vi "Acquisition Message Loop.vi"(8 "error in (no error)":errorcluster, 9 "queue out":refnum<queue>, 10 "Data Notifier":refnum<notifier>, 11 "Message Queues":T1) -> (0 "error out":errorcluster)   [LabVIEW 2018, in "Acquisition.lvlib"]
doc: "Message loop for handling messages pertaining to the acquisition of data from the hardware."
uses:
  Acquisition.lvlib
  support/Message Queue/Message Queue.lvlib
  Acquisition State.ctl
  support/Message Queue/Enqueue Message (Single).vi
  <vilib>/ErrorRing/Error Ring.xnode
  GlobalVariable/GlobalPowerByTime.vi
  GlobalVariable/Globalt0.vi
  GlobalVariable/GlobalLongueurOnde.vi
  GlobalVariable/GlobalDisconnected.vi
  GlobalVariable/GlobalPosXbyTime.vi
  GlobalVariable/GlobalPosYbyTime.vi
  GlobalVariable/GlobalProfileByTime.vi
  GlobalVariable/GlobalTimeStep.vi
  GlobalVariable/GlobalFirstRep.vi
  GlobalVariable/GlobalTensionByTime.vi
  GlobalVariable/GlobalTemperatureByTime.vi
  <vilib>/Utility/error.llb/Error Cluster From Error Code.vi
  support/Message Queue/Message Cluster.ctl
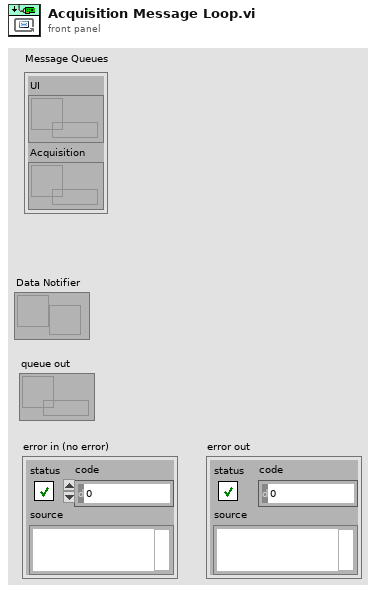
[diagram p1: front panel]
types:
  T1 = cluster{"UI":refnum<queue>, "Acquisition":refnum<queue>}
  T2 = typedef "Acquisition.lvlib/Acquisition State.ctl" = enum16{"Idle", "Acquiring"}
  T3 = enum16{"open", "replace", "create", "open or create", "replace or create", "replace or create with confirmation"}
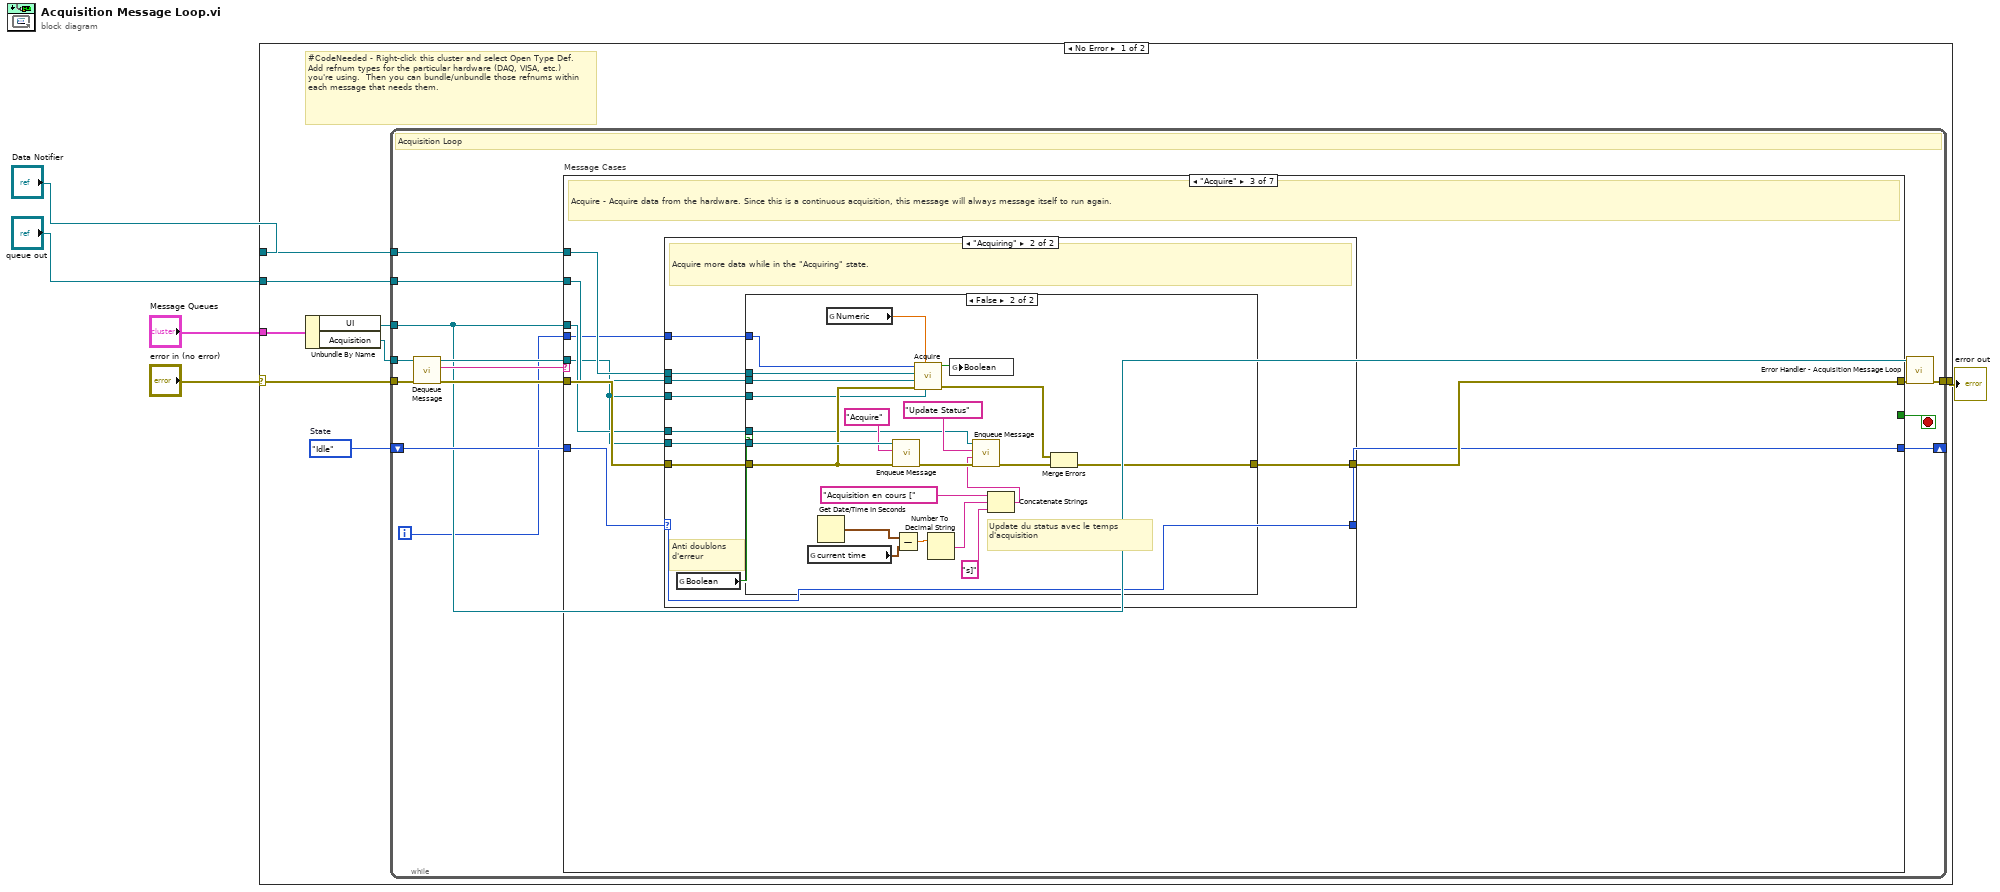
[diagram p0: block diagram]
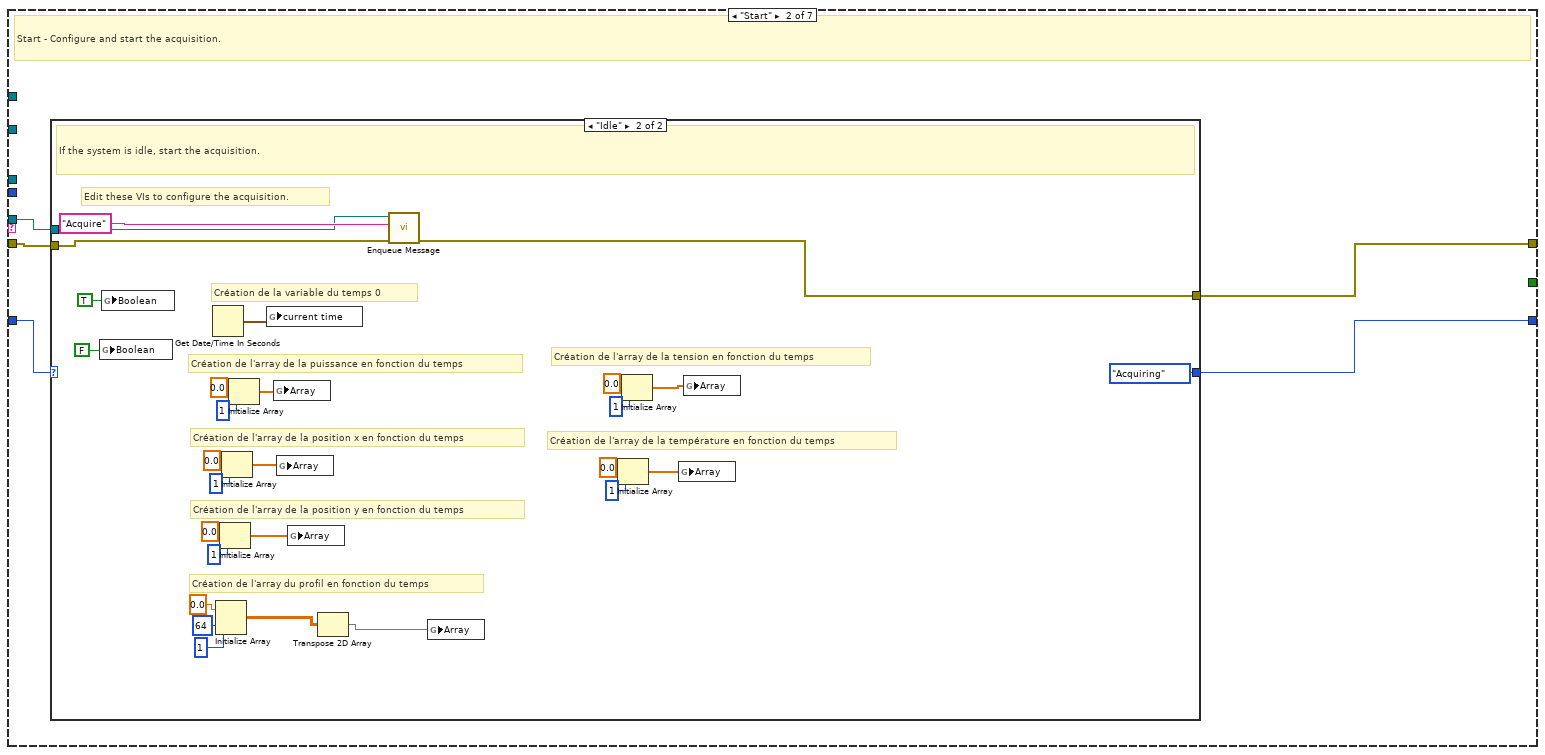
[diagram p3: hidden frame]
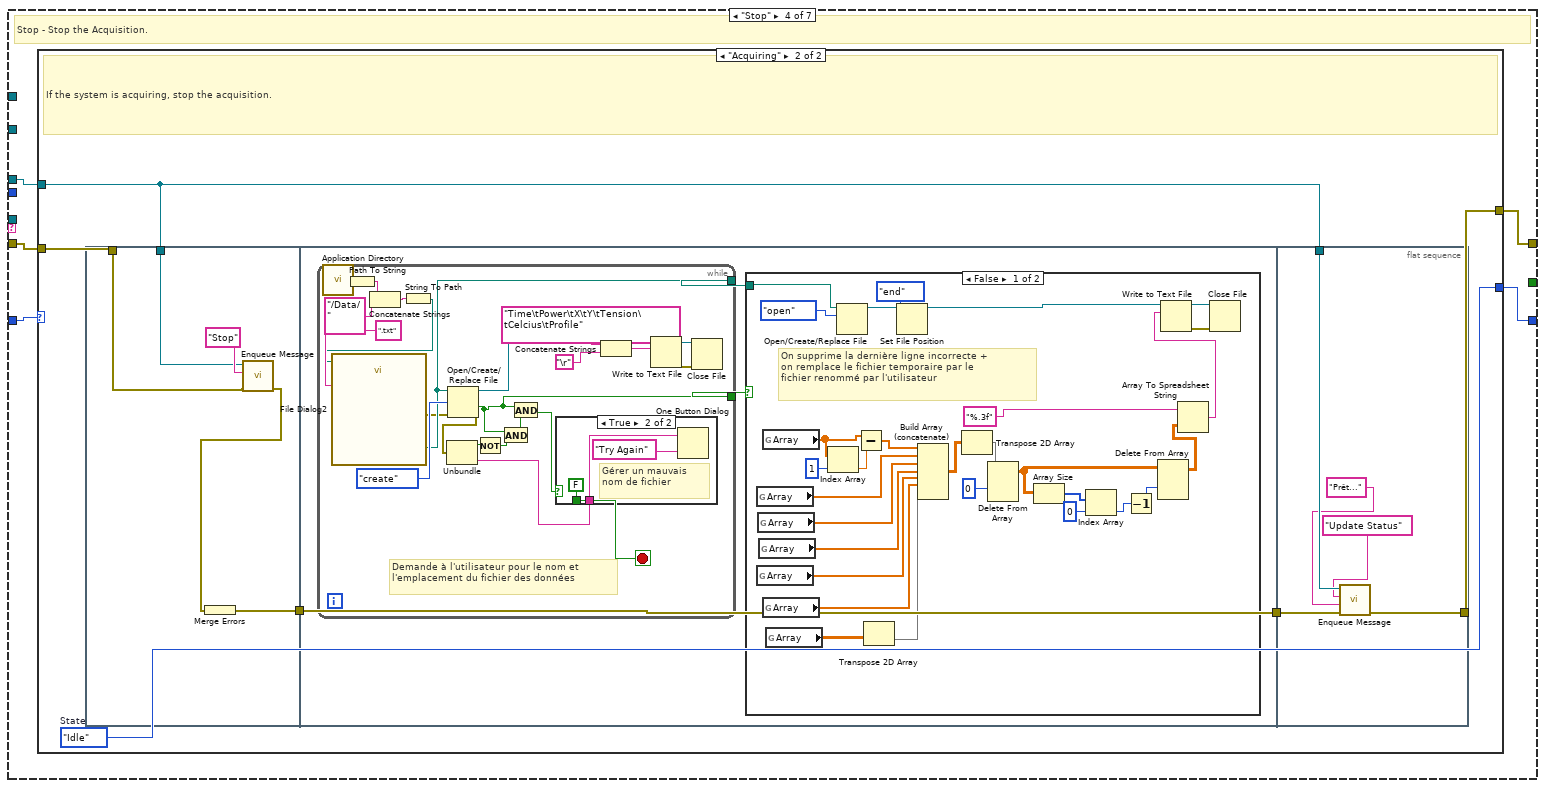
[diagram p7: hidden frame]
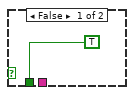
[diagram p10: hidden frame]
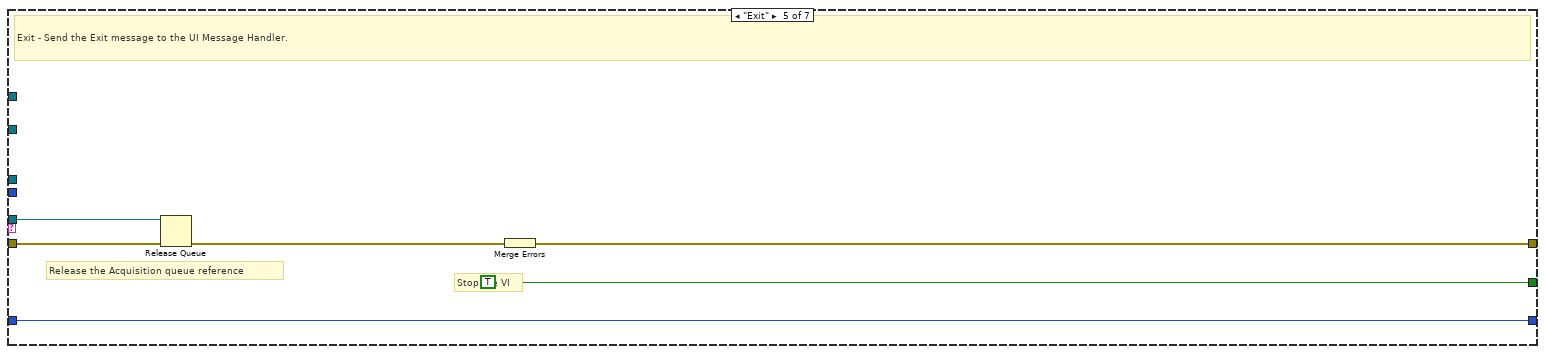
[diagram p11: hidden frame]
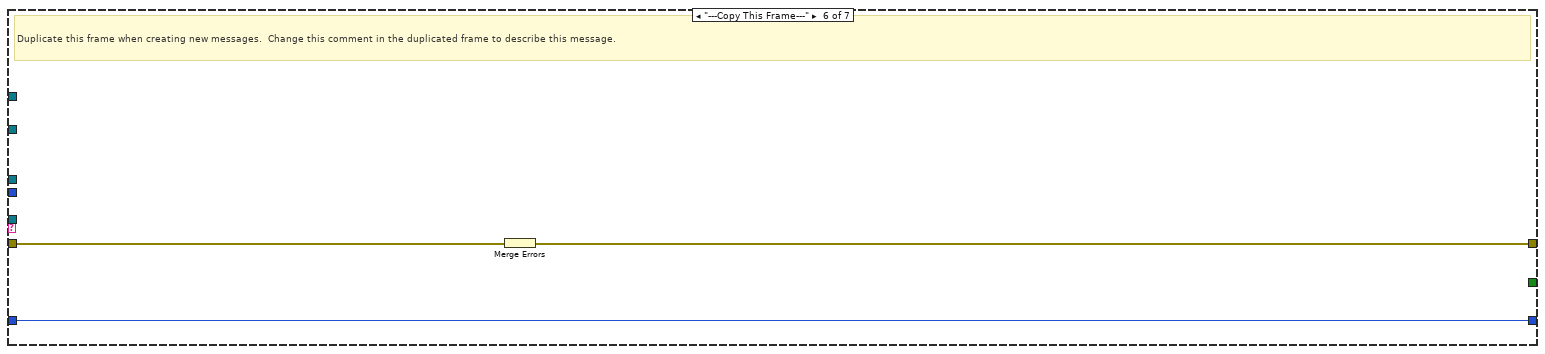
[diagram p12: hidden frame]
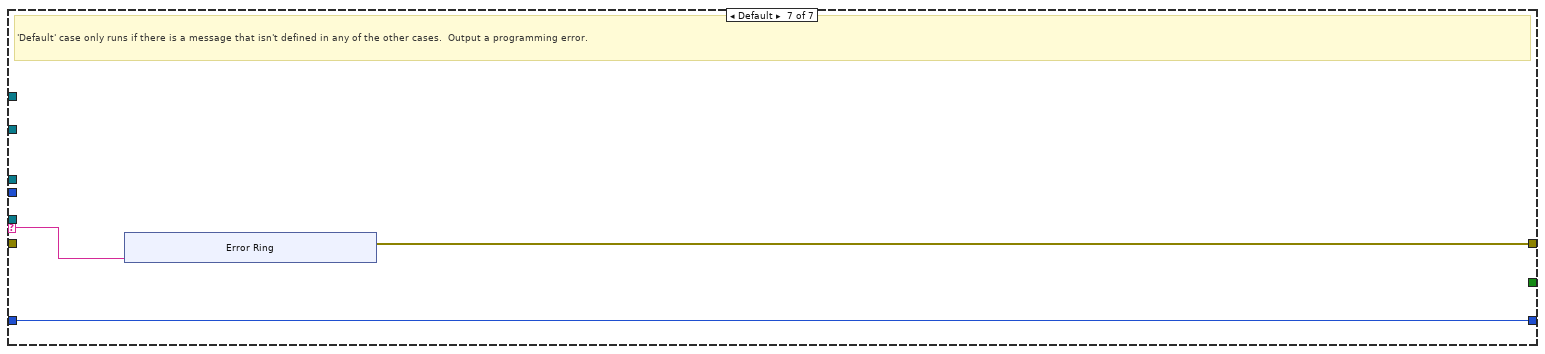
[diagram p13: hidden frame]
diagram:
  n1 = case shown="No Error" "error in (no error)" {
    selector: "error in (no error)" -> [w10 w210]
    tunnel: "Message Queues" -> [w13 _]
    tunnel: [w11 w210] -> w4
    tunnel: "Data Notifier" -> [w8 _]
    tunnel: "queue out" -> [w7 _]
    frame No Error {
      w6 = Acquisition_State."Idle"  # State
      # "#CodeNeeded - Right-click this cluster and select Open Type Def.  Add refnum types for the particular hardware (DAQ, VISA, etc.) you're using.  Then you can bundle/unbundle those refnums within each message that needs them."
      n2 = Unbundle By Name(w13) -> ("UI"=w9:refnum<queue>, "Acquisition"=w12:refnum<queue>)
      n3 = while {
        tunnel: w12 -> [w15]
        tunnel: w9 -> [w16]
        tunnel: w8 -> [w23]
        tunnel: w7 -> [w22]
        shift-right: [w20] -> _
        shift-left: w6 -> [w21]
        tunnel: w10 -> [w26]
        tunnel: [w19] -> w11
        i -> [w14]
        stop <- w27 stop-if-true
        # "Acquisition Loop"
        n4 = call "Dequeue Message.vi"("error in (no error)"=w26, "Message Queue"=w15) -> ("error out"=w25:errorcluster, "Message"=w24:string, "dup Message Queue"=w17:refnum<queue>)  [unwired: 6 in, 1 out]
        n5 = case "Message Cases" shown="\"Acquire\"" w24 {
          selector: w24 -> [_ _ _ _ _ _ w200]
          tunnel: w17 -> [_ w32 w66 _ w192 _ _]
          tunnel: w25 -> [w29 w33 w72 w112 w194 w199 _]
          tunnel: [w29 w34 w73 w110 w195 w198 w201] -> w18
          tunnel: [_ _ _ _ TRUE _ _] -> w27
          tunnel: w16 -> [_ _ w67 w111 _ _ _]
          tunnel: w23 -> [_ _ w71 _ _ _ _]
          tunnel: w22 -> [_ _ w70 _ _ _ _]
          tunnel: w21 -> [w28 w30 w68 w113 w191 w197 w202]
          tunnel: [w28 w31 w69 w109 w191 w197 w202] -> w20
          tunnel: w14 -> [_ _ w65 _ _ _ _]
          frame "Initialize" {
            # "Initialize  - Initialize is currently a no-op.  The hardware initialization takes place in the 'Start' message."
          }
          frame "Start" {
            # "Start - Configure and start the acquisition."
            n6 = case shown="\"Idle\"" w30 {
              selector: w30 -> [w35 _]
              tunnel: [w36 w60] -> w34
              tunnel: w33 -> [w36 w64]
              tunnel: w32 -> [_ w61]
              tunnel: [w35 Acquisition_State."Acquiring" ("Acquisition State")] -> w31
              frame "Acquiring" {
                # "The system is already acquiring. Ignore the \"Start\" message."
              }
              frame "Idle" {
                # "Création de l'array de la température en fonction du temps"
                # "Création de l'array de la tension en fonction du temps"
                # "Création de la variable du temps 0"
                # "Création de l'array du profil en fonction du temps"
                # "Création de l'array de la position y en fonction du temps"
                # "Création de l'array de la position x en fonction du temps"
                # "Création de l'array de la puissance en fonction du temps"
                # "Edit these VIs to configure the acquisition."
                # "If the system is idle, start the acquisition."
                n7 = global write "GlobalDisconnected.vi" "Boolean"(FALSE) -> ()
                n8 = global write "GlobalFirstRep.vi" "Boolean"(TRUE ("Boolean")) -> ()
                n9 = Get Date/Time In Seconds() -> (seconds since 1Jan1904=w43:timestamp)
                n10 = Initialize Array(0.0, 64 ("dimension size"), 1 ("dimension size")) -> (w56:dbl[][])
                n11 = Initialize Array(0.0, 1) -> (w57:dbl[])
                n12 = Initialize Array(0.0, 1) -> (w58:dbl[])
                n13 = Initialize Array(0.0, 1) -> (w59:dbl[])
                n14 = global write "Globalt0.vi" "current time"(w43) -> ()
                n15 = global write "GlobalPowerByTime.vi" "Array"(w59) -> ()
                n16 = global write "GlobalPosXbyTime.vi" "Array"(w58) -> ()
                n17 = global write "GlobalPosYbyTime.vi" "Array"(w57) -> ()
                n18 = Transpose 2D Array(2D array=w56) -> (transposed array=w55:dbl[][])
                n19 = call-poly "Enqueue Message.vi"("error in (no error)"=w64, "Message"="Acquire", "Message Queue"=w61) -> ("error out"=w60:errorcluster)  [unwired: 7 in, 1 out]
                n20 = global write "GlobalProfileByTime.vi" "Array"(w55) -> ()
                n21 = Initialize Array(0.0, 1) -> (w37:dbl[])
                n22 = Initialize Array(0.0, 1) -> (w38:dbl[])
                n23 = global write "GlobalTemperatureByTime.vi" "Array"(w37) -> ()
                n24 = global write "GlobalTensionByTime.vi" "Array"(w38) -> ()
              }
            }
          }
          frame "Acquire" {
            # "Acquire - Acquire data from the hardware. Since this is a continuous acquisition, this message will always message itself to run again."
            n25 = case shown="\"Acquiring\"" w68 {
              selector: w68 -> [w74 w81]
              tunnel: [w75 w85] -> w73
              tunnel: w66 -> [_ w84]
              tunnel: w72 -> [w75 w80]
              tunnel: w71 -> [_ w83]
              tunnel: w70 -> [_ w82]
              tunnel: [w74 w81] -> w69
              tunnel: w67 -> [_ w79]
              tunnel: w66 -> [_ w78]
              tunnel: w65 -> [_ w76]
              frame "Idle" {
                # "Ignore \"Acquire\" messages when the acquisition is idle."
              }
              frame "Acquiring" {
                # "Anti doublons\nd'erreur"
                # "Acquire more data while in the \"Acquiring\" state."
                n26 = global read "GlobalDisconnected.vi" "Boolean"() -> (w77:bool)
                n27 = case shown="False" w77 {
                  tunnel: [w86 w108] -> w85
                  tunnel: w84 -> [_ w107]
                  tunnel: w83 -> [_ w104]
                  tunnel: w82 -> [_ w103]
                  tunnel: w80 -> [w86 w102]
                  tunnel: w79 -> [_ w91]
                  tunnel: w78 -> [_ w90]
                  tunnel: w76 -> [_ w87]
                  frame True {
                  }
                  frame False {
                    # "Update du status avec le temps\nd'acquisition"
                    n28 = global read "Globalt0.vi" "current time"() -> (w97:timestamp)
                    n29 = Get Date/Time In Seconds() -> (seconds since 1Jan1904=w96:timestamp)
                    n30 = global read "GlobalLongueurOnde.vi" "Numeric"() -> (w89:dbl)
                    n31 = call-poly "Enqueue Message.vi"("error in (no error)"=w102, "Message"="Acquire", "Message Queue"=w107) -> ("error out"=w100:errorcluster)  [unwired: 7 in, 1 out]
                    n32 = Subtract(x=w96, y=w97) -> (x-y=w98:dbl)
                    n33 = call "Acquire.vi"("Acquisition"=w90, "Longueur d'onde"=w89, "error in (no error)"=w102, "Data Queue"=w103, "Data Notifier"=w104, "Loop Count"=w87) -> ("error out"=w106:errorcluster, "Disconnected"=w88:bool)  [unwired: 4 in]
                    n34 = Number To Decimal String(number=w98) -> (decimal integer string=w95:string)  [unwired: 1 in]
                    n35 = global write "GlobalDisconnected.vi" "Boolean"(w88) -> ()
                    n36 = Concatenate Strings("Acquisition en cours [", w95, "s]" ("string")) -> (w93:string)
                    n37 = call-poly "Enqueue Message.vi"("error in (no error)"=w100, "Message Data"=w93, "Message"="Update Status", "Message Queue"=w91) -> ("error out"=w101:errorcluster)  [unwired: 6 in, 1 out]
                    n38 = Merge Errors(w106, w101) -> (w108:errorcluster)
                  }
                }
              }
            }
          }
          frame "Stop" {
            # "Stop - Stop the Acquisition."
            n39 = case shown="\"Acquiring\"" w113 {
              selector: w113 -> [w115 _]
              tunnel: w112 -> [w114 w120]
              tunnel: w111 -> [_ w116]
              tunnel: [w114 w119] -> w110
              tunnel: [w115 w118] -> w109
              frame "Idle" {
                # "The system is already idle. Ignore the \"Stop\" message."
              }
              frame "Acquiring" {
                w118 = Acquisition_State."Idle"  # State
                # "If the system is acquiring, stop the acquisition."
                n40 = flat-sequence {
                  tunnel: [w126] -> w121
                  tunnel: w116 -> [w123]
                  tunnel: w120 -> [w122]
                  tunnel: w121 -> [w128]
                  tunnel: [w128] -> w117
                  tunnel: [w189] -> w119
                  tunnel: w117 -> [w190]
                  tunnel: w116 -> [w188]
                  frame #0 {
                    n41 = call-poly "Enqueue Message.vi"("error in (no error)"=w122, "Message"="Stop", "Message Queue"=w123) -> ("error out"=w125:errorcluster)  [unwired: 7 in, 1 out]
                    n42 = Merge Errors(w125) -> (w126:errorcluster)
                  }
                  frame #1 {
                    n43 = while {
                      tunnel: [w176] -> w129
                      tunnel: [w166] -> w127
                      stop <- w172 stop-if-true
                      # "Demande à l'utilisateur pour le nom et\nl'emplacement du fichier des données"
                      n44 = call <vilib>:"Application Directory.vi"() -> ("Application Directory"=w179:path)
                      n45 = Path To String(path=w179) -> (string=w180:string)
                      n46 = Concatenate Strings(w180, "/Data/") -> (w181:string)
                      n47 = String To Path(string=w181) -> (path=w165:path)
                      n48 = call "File Dialog2"("start path"=w165, "pattern (all files)"=".txt") -> ("selected path"=w176:path, "error out"=w174:errorcluster)  [unwired: 10 in, 2 out]
                      n49 = Open/Create/Replace File(file path (use dialog)=w176, error in=w174, operation (0:open)=T3."create") -> (refnum out=w161:refnum<file>, cancelled=w166:bool, error out=w171:errorcluster)  [unwired: 3 in]
                      n50 = Unbundle(w171) -> ("status"=w170:bool, "source"=w173:string)  [unwired: 1 out]
                      n51 = Not(x=w170) -> (.not. x?=w169:bool)
                      n52 = And(x=w166, y=w169) -> (x .and. y?=w168:bool)
                      n53 = And(x=w166, y=w168) -> (x .and. y?=w167:bool)
                      n54 = case shown="True" w167 {
                        tunnel: w173 -> [_ w185]
                        tunnel: [TRUE FALSE] -> w172
                        frame False {
                        }
                        frame True {
                          # "Gérer un mauvais \nnom de fichier"
                          n55 = One Button Dialog(message=w185, button name ("OK")="Try Again") -> ()  [unwired: 1 out]
                        }
                      }
                      n56 = Concatenate Strings("Time\tPower\tX\tY\tTension\tCelcius\tProfile", "\r") -> (w164:string)
                      n57 = Write to Text File(file (use dialog)=w161, text=w164) -> (refnum out=w160:refnum<file>, error out=w159:errorcluster)  [unwired: 2 in, 1 out]
                      n58 = Close File(refnum=w160, error in=w159) -> ()  [unwired: 2 out]
                    }
                    n59 = case shown="False" w127 {
                      tunnel: w129 -> [w152 _]
                      frame False {
                        # "On supprime la dernière ligne incorrecte + \non remplace le fichier temporaire par le \nfichier renommé par l'utilisateur"
                        n60 = global read "GlobalPowerByTime.vi" "Array"() -> (w151:dbl[])
                        n61 = global read "GlobalTensionByTime.vi" "Array"() -> (w131:dbl[])
                        n62 = global read "GlobalPosXbyTime.vi" "Array"() -> (w150:dbl[])
                        n63 = global read "GlobalPosYbyTime.vi" "Array"() -> (w149:dbl[])
                        n64 = global read "GlobalTimeStep.vi" "Array"() -> (w139:dbl[])
                        n65 = global read "GlobalTemperatureByTime.vi" "Array"() -> (w130:dbl[])
                        n66 = global read "GlobalProfileByTime.vi" "Array"() -> (w147:dbl[][])
                        n67 = Index Array(array=w139, index=1) -> (element=w140:dbl)
                        n68 = Open/Create/Replace File(file path (use dialog)=w152, operation (0:open)=T3."open") -> (refnum out=w156:refnum<file>)  [unwired: 4 in, 2 out]
                        n69 = Subtract(x=w139, y=w140) -> (x-y=w138:dbl[])
                        n70 = Transpose 2D Array(2D array=w147) -> (transposed array=w146:dbl[][])
                        n71 = Set File Position(refnum=w156, from (0:start)=enum16{"start", "end", "current"}."end") -> (refnum out=w158:refnum<file>)  [unwired: 2 in, 1 out]
                        n72 = Build Array (concatenate)(w138, w151, w150, w149, w131, w130, w146) -> (w148:dbl[][])
                        n73 = Transpose 2D Array(2D array=w148) -> (transposed array=w142:dbl[][])
                        n74 = Delete From Array(array=w142, index (row)=0) -> (array with subset deleted=w133:dbl[][])  [unwired: 2 in, 1 out]
                        n75 = Array Size(array=w133) -> (size(s)=w137:i32[])
                        n76 = Index Array(array=w137, index=0) -> (element=w135:i32)
                        n77 = Decrement(x=w135) -> (x-1=w134:i32)
                        n78 = Delete From Array(array=w133, index (row)=w134) -> (array with subset deleted=w132:dbl[][])  [unwired: 2 in, 1 out]
                        n79 = Array To Spreadsheet String(array=w132, 3:"%.3f" ("format string")) -> (spreadsheet string=w157:string)  [unwired: 1 in]
                        n80 = Write to Text File(file (use dialog)=w158, text=w157) -> (refnum out=w145:refnum<file>, error out=w144:errorcluster)  [unwired: 2 in, 1 out]
                        n81 = Close File(refnum=w145, error in=w144) -> ()  [unwired: 2 out]
                      }
                      frame True {
                      }
                    }
                  }
                  frame #2 {
                    n82 = call-poly "Enqueue Message.vi"("error in (no error)"=w190, "Message Data"="Prêt...", "Message"="Update Status", "Message Queue"=w188) -> ("error out"=w189:errorcluster)  [unwired: 6 in, 1 out]
                  }
                }
              }
            }
          }
          frame "Exit" {
            # "Release the Acquisition queue reference"
            # "Stop the VI"
            # "Exit - Send the Exit message to the UI Message Handler."
            n83 = Release Queue(queue=w192, error in (no error)=w194) -> (error out=w193:errorcluster)  [unwired: 1 in, 2 out]
            n84 = Merge Errors(w193) -> (w195:errorcluster)
          }
          frame "---Copy This Frame---" {
            # "Duplicate this frame when creating new messages.  Change this comment in the duplicated frame to describe this message."
            n85 = Merge Errors(w199) -> (w198:errorcluster)
          }
          frame Default {
            # "'Default' case only runs if there is a message that isn't defined in any of the other cases.  Output a programming error."
            n86 = xnode "Error Ring"("parameter 0"=w200) -> ("error out"=w201:errorcluster)
          }
        }
        n87 = call "Error Handler - Acquisition Message Loop.vi"("error in (no error)"=w18, "Message Queue"=w16) -> ("dup error in"=w19:errorcluster)  [unwired: 8 in, 1 out]
      }
    }
    frame Error {
    }
  }
  "error out" <- w4
